vi "UHR-Fleezers Control (host) - 10.4.vi"() -> ()   [LabVIEW 2011] (continued)
            n1668 = Sign(1:w3670) -> (0:w3669:dbl)
            n1669 = Compound Arithmetic op=MULTIPLY(w3670, "MCL Step Position Ratio", "MCL/AOM Scale Tweak") -> (w3674:dbl)
            n1670 = Negate(x=w3669) -> (-x=w3666:dbl)
            n1671 = Multiply(x=w3666, y="MCL Step Increment (V_int)") -> (x*y=w3668:dbl)
            n1672 = Divide(x=w3674, y="MCL X Cal (nm/V)") -> (x/y=w3680:dbl)
            n1673 = Multiply(x=32767.0 ("y"), y=w3680) -> (x*y=w3686:dbl)
            n1674 = local read "Total Counts (ticks)"() -> (w3671:u32)
            n1675 = local read "Cycles/step (AOD)"() -> (w3682:u64)
            n1676 = local read "Scan steps (AOD)"() -> (w3683:u64)
            n1677 = Divide(x=w3686, y=10.0) -> (x/y=w3679:dbl)
            n1678 = Divide(x=w3679, y="MCL Step Increment (V_int)") -> (x/y=w3677:dbl)
            n1679 = Absolute Value(x=w3677) -> (abs(x)=w3665:dbl)
            n1680 = Compound Arithmetic op=MULTIPLY(w3683, w3682, w3671) -> (w3678:u64)
            n1681 = local write "wait to reset values"(w3693) -> ()
            n1682 = local write "MCL Scanning"(w3693) -> ()
            n1683 = Divide(x=w3678, y=w3665) -> (x/y=w3675:dbl)
            "MCL Count" <- w3675
            n1684 = xnode "Read/Write Control"("FPGA VI Reference In"=w3692, "error in"=w3691, "Scan steps (MCL)"=w3665, "Number of scans (MCL)"=w3687, "Cycles per step (MCL)"=u64 1, "Scan freq.  increment (MCL)"=w3668, "1D or 2D Scan?"=w3688, "MCL Scan Axis"=w3688, "Cont. Scan (MCL)"=w3688, "MCL count"=w3675) -> ("FPGA VI Reference Out"=w3690:T19, "error out"=w3689:errorcluster)
            n1685 = xnode "Read/Write Control"("FPGA VI Reference In"=w3690, "error in"=w3689, "AI to FIFO"=w3693, "APD to FIFO"=w3693, "Start scan"=w3693, "Start scan (MCL)"=w3693) -> ("FPGA VI Reference Out"=w3695:T19, "error out"=w3694:errorcluster)
          }
        }
        "Raster Scanning..." <- TRUE ("Scanning...")
      }
    }
    n1686 = And(x="Save scans", y=w2773) -> (x .and. y?=w2819:bool)
    n1687 = Compound Arithmetic op=OR("Start MCL Scan", "Confocal Image", "Confocal Linescan") -> (w2771:bool)
    n1688 = And(x="Save Data (MCL)", y=w2771) -> (x .and. y?=w2818:bool)
    n1689 = case "Start MCL raster scan" shown="True" w2771 {
      tunnel: w2821 -> [w3266 w3282]
      tunnel: w2820 -> [w3265 w3281]
      tunnel: [w3266 w3277] -> w2660
      tunnel: [w3265 w3276] -> w2659
      tunnel: [FALSE w3275] -> w2804
      tunnel: "Start MCL Scan" -> [_ w3270]
      tunnel: "Confocal Image" -> [_ w3269]
      tunnel: "Confocal Linescan" -> [_ _]
      frame False {
      }
      frame True {
        w3275 = TRUE
        n1690 = case shown="True" "Restart DMA? (MCL)" {
          tunnel: [w3327 w3329] -> w3280
          tunnel: [w3326 w3328] -> w3279
          tunnel: w3282 -> [w3327 w3332]
          tunnel: w3281 -> [w3326 w3331]
          frame False {
          }
          frame True {
            n1691 = call "reset FPGA DMA.vi"("error in"=w3331, "FPGA VI Reference In"=w3332) -> ("error out"=w3328:errorcluster, "FPGA VI Reference Out"=w3329:T19)
            n1692 = local write "Overflow (data lost)"(FALSE ("Overflow (data lost)")) -> ()
          }
        }
        n1693 = case shown="False" w3270 {
          selector: w3270 -> [_ w3286]
          tunnel: w3269 -> [w3285 _]
          tunnel: [w3285 w3286] -> w3268
          frame False {
            n1694 = property on="2D or 1D Scan" class="Bool (strict)"("Val(Sgnl)"=w3285) -> ()  [unwired: 2 in, 2 out]
            n1695 = property on="Confocal Image" class="Bool (strict)"("Value"=FALSE ("Start Confocal Map")) -> ()  [unwired: 2 in, 2 out]
          }
          frame True {
          }
        }
        n1696 = local write "MCL Scanning"(w3275) -> ()
        n1697 = local read "AO1"() -> (w3272:dbl)
        n1698 = local read "AO2"() -> (w3271:dbl)
        n1699 = case shown="True" "Center Scan" {
          tunnel: w3280 -> [w3293 w3325]
          tunnel: w3279 -> [w3292 w3324]
          tunnel: [w3291 w3323] -> w3277
          tunnel: [w3290 w3322] -> w3276
          tunnel: [w3288 w3309] -> w3274
          tunnel: [w3287 w3308] -> w3273
          tunnel: w3272 -> [w3288 w3314]
          tunnel: w3271 -> [w3287 w3317]
          tunnel: w3268 -> [_ _]
          frame False {
            w3289 = TRUE ("AI to FIFO")
            n1700 = xnode "Read/Write Control"("FPGA VI Reference In"=w3293, "error in"=w3292, "AI to FIFO"=w3289, "APD to FIFO"=w3289, "Start scan (MCL)"=w3289) -> ("FPGA VI Reference Out"=w3291:T19, "error out"=w3290:errorcluster)
          }
          frame True {
            w3321 = TRUE ("AI to FIFO")
            n1701 = local read "Scan steps (MCL)"() -> (w3300:u64)
            n1702 = local read "Scan lines (y)"() -> (w3296:u64)
            n1703 = local read "Fast Scan Dir"() -> (w3307:bool)
            n1704 = local read "Actual MCL Inc (V)"() -> (w3297:dbl)
            n1705 = Decrement(x=w3296) -> (x-1=w3295:u64)
            n1706 = Decrement(x=w3300) -> (x-1=w3299:u64)
            n1707 = Multiply(x=w3297, y=w3295) -> (x*y=w3294:dbl)
            n1708 = Divide(x=w3294, y=2.0) -> (x/y=w3304:dbl)
            n1709 = Multiply(x=w3297, y=w3299) -> (x*y=w3298:dbl)
            n1710 = Divide(x=w3298, y=2.0) -> (x/y=w3303:dbl)
            n1711 = Select(t=w3303, s=w3307, f=w3304) -> (s? t:f=w3302:dbl)
            n1712 = Select(t=w3304, s=w3307, f=w3303) -> (s? t:f=w3306:dbl)
            n1713 = Subtract(x=w3314, y=w3306) -> (x-y=w3305:dbl)
            n1714 = Subtract(x=w3317, y=w3302) -> (x-y=w3301:dbl)
            n1715 = local read "2D or 1D Scan"() -> (w3319:bool)
            n1716 = Not(x=w3307) -> (.not. x?=w3313:bool)
            n1717 = Not(x=w3319) -> (.not. x?=w3315:bool)
            n1718 = And(x=w3307, y=w3315) -> (x .and. y?=w3316:bool)
            n1719 = And(x=w3315, y=w3313) -> (x .and. y?=w3318:bool)
            n1720 = Select(t=w3317, s=w3318, f=w3301) -> (s? t:f=w3308:dbl)
            n1721 = Select(t=w3314, s=w3316, f=w3305) -> (s? t:f=w3309:dbl)
            n1722 = call "Volt to I16.vi"("Voltage In"=w3309) -> ("I16 Voltage Out"=w3312:i16)
            n1723 = call "Volt to I16.vi"("Voltage In"=w3308) -> ("I16 Voltage Out"=w3311:i16)
            n1724 = xnode "Read/Write Control"("FPGA VI Reference In"=w3325, "error in"=w3324, "AI to FIFO"=w3321, "APD to FIFO"=w3321, "Start scan (MCL)"=w3321, "AO1"=w3312, "AO2"=w3311) -> ("FPGA VI Reference Out"=w3323:T19, "error out"=w3322:errorcluster)
          }
        }
        "Initial Y" <- w3274
        "Initial X" <- w3273
        n1725 = local write "Tab Control 6"(T3."Imaging" ("Tab Control 6")) -> ()
        "wait to reset values" <- w3275
      }
    }
    n1726 = local read "Trap Pos Elements/DMA read"() -> (w2656:u32)
    n1727 = local read "Trap AI Elements/DMA read"() -> (w2732:u32)
    n1728 = local read "APD Elements/DMA read"() -> (w2697:u32)
    n1729 = xnode "Get APD Data"("FPGA VI Reference In"=w2660, "error in"=w2659, "Number of Elements"=w2697, "Timeout (ms)"=-1) -> ("Data"=w2696:u32[], "Elements Remaining"=→"APD FIFO Elements Remaining":u32)  [unwired: 2 out]
    n1730 = xnode "Invoke Method"("FPGA VI Reference In"=w2660, "error in"=w2659, "Number of Elements"=w2656, "Timeout (ms)"=-1) -> ("Data"=w2619:u16[], "Elements Remaining"=→"Trap Pos FIFO El Remaining":u32)  [unwired: 2 out]
    n1731 = xnode "Get Trap Data"("FPGA VI Reference In"=w2660, "error in"=w2659, "Number of Elements"=w2732, "Timeout (ms)"=-1 ("Timeout")) -> ("FPGA VI Reference Out"=w2553:T19, "error out"=w2552:errorcluster, "Data"=w2620:i16[], "Elements Remaining"=w2865:u32)
    "FIFO El. Rem." <- w2865
    n1732 = local read "Trap AI FIFO Depth"() -> (w2867:u32)
    n1733 = Subtract(x=w2867, y=w2732) -> (x-y=w2866:u32)
    n1734 = Decimate 1D Array(w2619) -> (w2616:u16[], w2618:u16[], w2617:u16[])
    n1735 = Divide(x=w2865, y=w2866) -> (x/y=w2864:dbl)
    "Buffer Status" <- w2864
    n1736 = To Unsigned Long Integer(number=w2616) -> (unsigned 32bit integer=w2615:u32[])
    n1737 = Join Numbers(hi=w2618, lo=w2617) -> ((hi.lo)=w2614:u32[])
    n1738 = Equal?(x=w2864, y=1.0) -> (x = y?=w2862:bool)
    n1739 = Join Numbers(hi=w2615, lo=w2614) -> ((hi.lo)=w2608:u64[])
    n1740 = call "IR AOM word to freq - vec.vi"("Frequency Word In (double vec)"=w2608) -> ("Frequency Out"=w2655:dbl[])
    n1741 = case "Alert buffer overflow" shown="True" w2862 {
      frame False {
      }
      frame True {
        n1742 = call <vilib>:"Beep.vi"() -> ()  [unwired: 3 in, 9 out]
        "Overflow (data lost)" <- TRUE ("Overflow (data lost)")
      }
    }
    n1743 = Decimate 1D Array(w2655) -> (w2654:dbl[], w2653:dbl[])
    n1744 = Build Array(w2654, w2653) -> (w2652:dbl[][])
    n1745 = local read "Trap Sets"() -> (w2731:u32)
    n1746 = case "Deinterlace trap data, average down PSD" shown="2" w2731 {
      tunnel: w2620 -> [w3362 w3427]
      tunnel: [w3359 w3424] -> w2724
      tunnel: [w3362 w3426] -> w2611
      tunnel: "Detector Type" -> [w3361 w3422]
      tunnel: [w3360 w3425] -> w2723
      tunnel: [w3358 w3423] -> w2839
      frame 1, Default {
        n1747 = Divide(x=w3362, y=3276.7) -> (x/y=w3363:dbl[])
        n1748 = Decimate 1D Array(w3363) -> (w3372:dbl[], w3371:dbl[], w3370:dbl[], w3369:dbl[], w3368:dbl[], w3367:dbl[], w3366:dbl[], w3365:dbl[])
        n1749 = case shown="\"IR-QPD + PSD + FB-QPD position\"" w3361 {
          tunnel: w3372 -> [w3396 w3421]
          tunnel: w3371 -> [w3395 w3420]
          tunnel: w3370 -> [w3380 w3398]
          tunnel: w3369 -> [w3381 w3408]
          tunnel: w3368 -> [w3394 w3419]
          tunnel: w3367 -> [w3393 w3418]
          tunnel: w3366 -> [w3377 w3399]
          tunnel: w3365 -> [w3376 w3397]
          tunnel: [w3375 w3405] -> w3360
          tunnel: [w3374 w3404] -> w3359
          tunnel: [w3373 w3403] -> w3358
          frame "IR-QPD + PSD + FB-QPD", Default {
            w3373 = 0  # Channel pattern
            n1750 = Divide(x=w3396, y=w3381) -> (x/y=w3383:dbl[])
            n1751 = Divide(x=w3395, y=w3381) -> (x/y=w3382:dbl[])
            n1752 = Divide(x=w3394, y=w3377) -> (x/y=w3379:dbl[])
            n1753 = Divide(x=w3393, y=w3376) -> (x/y=w3378:dbl[])
            n1754 = Build Array(w3383, w3382, w3381, w3380, w3379, w3378, w3377, w3376) -> (w3374:dbl[][])
            n1755 = Bundle("T1 Y", "T1 X", "T1 Sum", "FB Sum", "PSD Y", "PSD X", "PSD Y Sum", "PSD X Sum") -> (w3392:T40)  [unwired: 1 out]
            n1756 = Cluster To Array(cluster=w3392) -> (array=w3375:string[])
          }
          frame "IR-QPD + PSD + FB-QPD position" {
            w3403 = 3  # Channel pattern
            n1757 = Negate(x=w3399) -> (-x=w3400:dbl[])
            n1758 = Divide(x=w3421, y=w3408) -> (x/y=w3410:dbl[])
            n1759 = Divide(x=w3420, y=w3408) -> (x/y=w3409:dbl[])
            n1760 = Divide(x=w3419, y=w3399) -> (x/y=w3407:dbl[])
            n1761 = Divide(x=w3418, y=w3400) -> (x/y=w3406:dbl[])
            n1762 = Build Array(w3410, w3409, w3408, w3397, w3398, w3407, w3406, w3399) -> (w3404:dbl[][])
            n1763 = Bundle("T1 Y", "T1 X", "T1 Sum", "FB X", "FB Sum", "PSD Y", "PSD X", "PSD Y Sum") -> (w3417:T40)  [unwired: 1 out]
            n1764 = Cluster To Array(cluster=w3417) -> (array=w3405:string[])
          }
        }
      }
      frame 2 {
        n1765 = case shown="\"IR-QPD + PSD + FB-QPD X position\"" w3422 {
          tunnel: w3427 -> [w3489 w3556 w3627]
          tunnel: [w3428 w3547 w3558] -> w3426
          tunnel: [w3455 w3538 w3605] -> w3425
          tunnel: [w3454 w3501 w3572] -> w3424
          tunnel: [w3448 w3536 w3603] -> w3423
          frame "IR-QPD + PSD + FB-QPD", Default {
            w3448 = 1  # Channel pattern
            # "time average x2 the 4th signal and the 4 psd signals (detection laser)"
            # "deinterlace 3 signals from qpd"
            n1766 = Decimate 1D Array(w3489) -> (w3488:i16[], w3487:i16[], w3453:i16[], w3486:i16[], w3476:i16[], w3474:i16[], w3473:i16[], w3471:i16[])
            n1767 = Decimate 1D Array(w3453) -> (w3452:i16[], w3451:i16[])
            n1768 = Decimate 1D Array(w3488) -> (w3485:i16[], w3457:i16[])
            n1769 = Decimate 1D Array(w3487) -> (w3484:i16[], w3482:i16[])
            n1770 = Decimate 1D Array(w3486) -> (w3483:i16[], w3481:i16[])
            n1771 = call "downsample 1D array - double.vi"("Ave N"=2.0, "Array In"=w3476) -> ("Array Out"=w3475:dbl[])  [unwired: 1 out]
            n1772 = call "downsample 1D array - double.vi"("Ave N"=2.0, "Array In"=w3474) -> ("Array Out"=w3456:dbl[])  [unwired: 1 out]
            n1773 = call "downsample 1D array - double.vi"("Ave N"=2.0, "Array In"=w3473) -> ("Array Out"=w3472:dbl[])  [unwired: 1 out]
            n1774 = call "downsample 1D array - double.vi"("Ave N"=2.0, "Array In"=w3471) -> ("Array Out"=w3470:dbl[])  [unwired: 1 out]
            n1775 = Interleave 1D Arrays(w3485, w3484, w3483, w3457, w3482, w3481, w3452, w3451, w3475, w3456, w3472, w3470) -> (w3469:dbl[])
            n1776 = Divide(x=w3469, y=3276.7) -> (x/y=w3468:dbl[])
            n1777 = Decimate 1D Array(w3468) -> (w3467:dbl[], w3466:dbl[], w3465:dbl[], w3464:dbl[], w3463:dbl[], w3462:dbl[], w3450:dbl[], w3449:dbl[], w3461:dbl[], w3460:dbl[], w3459:dbl[], w3458:dbl[])
            n1778 = Divide(x=w3467, y=w3465) -> (x/y=w3435:dbl[])
            n1779 = Divide(x=w3466, y=w3465) -> (x/y=w3434:dbl[])
            n1780 = Divide(x=w3464, y=w3462) -> (x/y=w3433:dbl[])
            n1781 = Divide(x=w3463, y=w3462) -> (x/y=w3432:dbl[])
            n1782 = Divide(x=w3461, y=w3459) -> (x/y=w3431:dbl[])
            n1783 = Divide(x=w3460, y=w3458) -> (x/y=w3430:dbl[])
            n1784 = Build Array(w3435, w3434, w3465, w3433, w3432, w3462, w3450, w3449, w3431, w3430, w3459, w3458) -> (w3454:dbl[][])
            n1785 = Bundle("T1 Y", "T1 X", "T1 Sum", "T2 Y", "T2 X", "T2 Sum", "T1 FB Sum", "T2 FB Sum", "PSD Y", "PSD X", "PSD Y Sum", "PSD X Sum") -> (w3436:T41)  [unwired: 1 out]
            n1786 = To Word Integer(number=w3469) -> (16bit integer=w3428:i16[])
            n1787 = Cluster To Array(cluster=w3436) -> (array=w3455:string[])
          }
          frame "IR-QPD + PSD + FB-QPD X position" {
            w3536 = 2  # Channel pattern
            # "time average x2 the 3 psd signals (detection laser)"
            # "deinterlace 3 signals from qpds"
            n1788 = Decimate 1D Array(w3556) -> (w3555:i16[], w3554:i16[], w3537:i16[], w3553:i16[], w3499:i16[], w3496:i16[], w3493:i16[], w3524:i16[])
            n1789 = Decimate 1D Array(w3537) -> (w3522:i16[], w3520:i16[])
            n1790 = Decimate 1D Array(w3555) -> (w3552:i16[], w3539:i16[])
            n1791 = Decimate 1D Array(w3554) -> (w3551:i16[], w3549:i16[])
            n1792 = Decimate 1D Array(w3553) -> (w3550:i16[], w3548:i16[])
            n1793 = Decimate 1D Array(w3524) -> (w3523:i16[], w3521:i16[])
            n1794 = call "downsample 1D array - I16.vi"("Ave N"=2.0, "Array In"=w3499) -> ("Array Out"=w3497:i16[])  [unwired: 1 in]
            n1795 = call "downsample 1D array - I16.vi"("Ave N"=2.0, "Array In"=w3493) -> ("Array Out"=w3491:i16[])  [unwired: 1 in]
            n1796 = call "downsample 1D array - I16.vi"("Ave N"=2.0, "Array In"=w3496) -> ("Array Out"=w3494:i16[])  [unwired: 1 in]
            n1797 = Interleave 1D Arrays(w3552, w3551, w3550, w3539, w3549, w3548, w3523, w3522, w3521, w3520, w3497, w3494, w3491) -> (w3547:i16[])
            n1798 = Divide(x=w3547, y=3276.7) -> (x/y=w3546:dbl[])
            n1799 = Decimate 1D Array(w3546) -> (w3545:dbl[], w3544:dbl[], w3543:dbl[], w3542:dbl[], w3541:dbl[], w3540:dbl[], w3512:dbl[], w3510:dbl[], w3509:dbl[], w3507:dbl[], w3506:dbl[], w3505:dbl[], w3502:dbl[])
            n1800 = Negate(x=w3502) -> (-x=w3500:dbl[])
            n1801 = Divide(x=w3506, y=w3502) -> (x/y=w3504:dbl[])
            n1802 = Divide(x=w3505, y=w3500) -> (x/y=w3503:dbl[])
            n1803 = Divide(x=w3545, y=w3543) -> (x/y=w3528:dbl[])
            n1804 = Divide(x=w3544, y=w3543) -> (x/y=w3527:dbl[])
            n1805 = Divide(x=w3542, y=w3540) -> (x/y=w3526:dbl[])
            n1806 = Divide(x=w3541, y=w3540) -> (x/y=w3525:dbl[])
            n1807 = Divide(x=w3512, y=w3510) -> (x/y=w3511:dbl[])
            n1808 = Divide(x=w3509, y=w3507) -> (x/y=w3508:dbl[])
            n1809 = Build Array(w3528, w3527, w3543, w3526, w3525, w3540, w3511, w3510, w3508, w3507, w3504, w3503, w3502) -> (w3501:dbl[][])
            n1810 = Bundle("T1 Y", "T1 X", "T1 Sum", "T2 Y", "T2 X", "T2 Sum", "T1 FB X", "T1 FB Sum", "T2 FB X", "T2 FB Sum", "PSD Y", "PSD X", "PSD Y Sum") -> (w3529:T42)  [unwired: 1 out]
            n1811 = Cluster To Array(cluster=w3529) -> (array=w3538:string[])
          }
          frame "IR-QPD + PSD + FB-QPD XY positions" {
            w3603 = 4  # Channel pattern
            # "time average x2 the 3 psd signals (detection laser)"
            # "deinterlace 3 signals from qpds"
            n1812 = Decimate 1D Array(w3627) -> (w3626:i16[], w3625:i16[], w3604:i16[], w3624:i16[], w3570:i16[], w3616:i16[], w3615:i16[], w3592:i16[])
            n1813 = Decimate 1D Array "Feedback Sum"(w3604) -> (w3588:i16[], w3586:i16[])
            n1814 = Decimate 1D Array "QPD Y"(w3626) -> (w3623:i16[], w3606:i16[])
            n1815 = Decimate 1D Array "QPD X"(w3625) -> (w3622:i16[], w3620:i16[])
            n1816 = Decimate 1D Array "Feedback Y"(w3570) -> (w3569:i16[], w3568:i16[])
            n1817 = Decimate 1D Array "QPD Sum"(w3624) -> (w3621:i16[], w3619:i16[])
            n1818 = Decimate 1D Array "Feedback X"(w3592) -> (w3589:i16[], w3587:i16[])
            n1819 = call "downsample 1D array - double.vi"("Ave N"=2.0, "Array In"=w3616) -> ("Array Out"=w3591:dbl[])  [unwired: 1 out]
            n1820 = call "downsample 1D array - double.vi"("Ave N"=2.0, "Array In"=w3615) -> ("Array Out"=w3590:dbl[])  [unwired: 1 out]
            n1821 = Interleave 1D Arrays(w3623, w3622, w3621, w3606, w3620, w3619, w3569, w3589, w3588, w3568, w3587, w3586, w3591, w3590) -> (w3614:dbl[])
            n1822 = Divide(x=w3614, y=3276.7) -> (x/y=w3613:dbl[])
            n1823 = Decimate 1D Array(w3613) -> (w3612:dbl[], w3611:dbl[], w3610:dbl[], w3609:dbl[], w3608:dbl[], w3607:dbl[], w3565:dbl[], w3579:dbl[], w3563:dbl[], w3564:dbl[], w3577:dbl[], w3561:dbl[], w3575:dbl[], w3573:dbl[])
            n1824 = Negate(x=w3573) -> (-x=w3571:dbl[])
            n1825 = Divide(x=w3575, y=w3571) -> (x/y=w3574:dbl[])
            n1826 = Divide(x=w3564, y=w3561) -> (x/y=w3560:dbl[])
            n1827 = Divide(x=w3565, y=w3563) -> (x/y=w3562:dbl[])
            n1828 = Divide(x=w3612, y=w3610) -> (x/y=w3596:dbl[])
            n1829 = Divide(x=w3611, y=w3610) -> (x/y=w3595:dbl[])
            n1830 = Divide(x=w3609, y=w3607) -> (x/y=w3594:dbl[])
            n1831 = Divide(x=w3608, y=w3607) -> (x/y=w3593:dbl[])
            n1832 = Divide(x=w3579, y=w3563) -> (x/y=w3578:dbl[])
            n1833 = Divide(x=w3577, y=w3561) -> (x/y=w3576:dbl[])
            n1834 = Build Array(w3596, w3595, w3610, w3594, w3593, w3607, w3562, w3578, w3563, w3560, w3576, w3561, w3574, w3573) -> (w3572:dbl[][])
            n1835 = Bundle("T1 Y", "T1 X", "T1 Sum", "T2 Y", "T2 X", "T2 Sum", "T1 FB Y", "T1 FB X", "T1 FB Sum", "T2 FB Y", "T2 FB X", "T2 FB Sum", "PSD X", "PSD Y Sum") -> (w3559:T43)  [unwired: 1 out]
            n1836 = To Word Integer(number=w3614) -> (16bit integer=w3558:i16[])
            n1837 = Cluster To Array(cluster=w3559) -> (array=w3605:string[])
          }
        }
      }
    }
    "AI labels" <- w2723
    n1838 = Decimate 1D Array(w2696) -> (w2721:u32[], w2664:u32[])
    n1839 = local read "DMA Update Period (s)"() -> (w2733:dbl)
    n1840 = Build Array(w2721, w2664) -> (w2801:u32[][])
    n1841 = local read "Data Period (s)"() -> (w2570:dbl)
    n1842 = local read "BD 1 Frequency 2 (MHz)"() -> (w2603:dbl)
    n1843 = local read "BD 1 Frequency 1 (MHz)"() -> (w2604:dbl)
    n1844 = Decimate 1D Array(w2611) -> (w2635:i16[], w2634:i16[], w2632:i16[], w2631:i16[])  [unwired: 9 out]
    n1845 = To Double Precision Float(number=w2801) -> (double precision float=w2802:dbl[][])
    n1846 = local read "APD Integration Time (s)"() -> (w2677:dbl)
    n1847 = Multiply(x=w2570, y="Trap Pos. Disp. Downsample") -> (x*y=w2568:dbl)
    n1848 = Divide(x=w2635, y=w2634) -> (x/y=w2636:dbl[])
    n1849 = Divide(x=w2632, y=w2631) -> (x/y=w2633:dbl[])
    n1850 = feedback #4(0.0) -> (w2649:dbl)
    n1851 = Add(x=w2733, y=w2649) -> (x+y=w2841:dbl)
    n1852 = feedback-in #4(w2841) -> ()
    n1853 = local read "AOM X Cal (nm/MHz)"() -> (w2601:dbl)
    n1854 = To Time Stamp(1:w2649) -> (0:w2648:timestamp)
    n1855 = Split 1D Array(array=w2636, index="N El. to Ave.") -> (second subarray=w2639:dbl[])  [unwired: 1 out]
    n1856 = Split 1D Array(array=w2633, index="N El. to Ave.") -> (second subarray=w2638:dbl[])  [unwired: 1 out]
    n1857 = Multiply(x=w2570, y="Trap Disp. Downsample") -> (x*y=w2650:dbl)
    "Display Period (s)" <- w2650
    n1858 = for "Trap AI" {
      tunnel: [w3357] -> w2835 mode=indexing
      tunnel: w2648 -> [w3347]
      tunnel: "Trap Disp. Downsample" -> [w3355]
      tunnel: w2724 -> [w3353] mode=indexing
      tunnel: w2570 -> [w3352]
      tunnel: w2723 -> [w3351] mode=indexing
      tunnel: w2647 -> [w3350]
      tunnel: [w3349] -> w2688 mode=indexing
      tunnel: w2650 -> [w3348]
      workers-P: _ -> [_]
      n1859 = Bundle By Name("Y"=w3353, "dt"=w3352) -> (w3354:waveform(dbl))  [unwired: 1 out]
      n1860 = Set Waveform Attribute(5:w3351, 6:w3350, 7:w3354) -> (3:w3349:waveform(dbl))  [unwired: 1 in, 2 out]
      n1861 = call "downsample 1D array - double.vi"("Ave N"=w3355, "Array In"=w3353) -> ("Array Out"=w3356:dbl[])  [unwired: 1 out]
      n1862 = Bundle By Name(cluster=w3349, "t0"=w3347, "Y"=w3356, "dt"=w3348) -> (w3357:waveform(dbl))
    }
    n1863 = Bundle("BD 1 Frequency 1 (MHz)"=w2604, "BD 1 Frequency 2 (MHz)"=w2603) -> (w2605:T44)  [unwired: 1 out]
    n1864 = call <vilib>:"Mean.vi"("X"=w2638) -> ("mean"=w2626:dbl)  [unwired: 1 out]
    n1865 = call <vilib>:"Mean.vi"("X"=w2639) -> ("mean"=w2627:dbl)  [unwired: 1 out]
    n1866 = Reciprocal(x=w2650) -> (1/x=→"Trap Disp. Freq. (Hz)":dbl)
    n1867 = Cluster To Array(cluster=w2605) -> (array=w2602:dbl[])
    n1868 = local read "Trap X AI1 (DMA)"() -> (w2637:T13)
    n1869 = local read "Data points/scans (MCL)"() -> (w2813:dbl)
    n1870 = To Fixed-Point(number=w2626) -> (fixed-point=w2624:fxp<+/-,16,1>)  [unwired: 1 in]
    n1871 = To Fixed-Point(number=w2627) -> (fixed-point=w2625:fxp<+/-,16,1>)  [unwired: 1 in]
    n1872 = Bundle("Trap 1 Pos.", "Trap 2 Pos.") -> (w2646:cluster{string, string})  [unwired: 1 out]
    n1873 = Bundle By Name(cluster=w2637, "Set 1"=w2625, "Set 2"=w2624) -> (→"Trap X AI1 (DMA)":T13)
    n1874 = Cluster To Array(cluster=w2646) -> (array=w2643:string[])
    n1875 = Bundle("APD 1", "APD 2") -> (w2834:cluster{string, string})  [unwired: 1 out]
    n1876 = Select(t=-1.0, s="Negate Y Axis", f=1.0) -> (s? t:f=w2587:dbl)
    n1877 = for "Trap Position" {
      tunnel: w2652 -> [w2996] mode=indexing
      tunnel: "Trap Pos. Disp. Downsample" -> [w2995]
      tunnel: w2568 -> [w2993]
      tunnel: w2648 -> [w2992]
      tunnel: w2647 -> [w2990]
      tunnel: w2643 -> [w2989] mode=indexing
      tunnel: [w2988] -> w2557 mode=indexing
      tunnel: w2602 -> [w2986] mode=indexing
      tunnel: w2601 -> [w2984]
      tunnel: w2587 -> [w2983]
      n1878 = call "downsample 1D array - double.vi"("Ave N"=w2995, "Array In"=w2996) -> ("Array Out"=w2994:dbl[])  [unwired: 1 out]
      n1879 = Subtract(x=w2994, y=w2986) -> (x-y=w2987:dbl[])
      n1880 = Multiply(x=w2984, y=w2987) -> (x*y=w2985:dbl[])
      n1881 = Multiply(x=w2983, y=w2985) -> (x*y=w2982:dbl[])
      n1882 = Bundle By Name("Y"=w2982, "dt"=w2993, "t0"=w2992) -> (w2991:waveform(dbl))  [unwired: 1 out]
      n1883 = Set Waveform Attribute(5:w2989, 6:w2990, 7:w2991) -> (3:w2988:waveform(dbl))  [unwired: 1 in, 2 out]
    }
    n1884 = Cluster To Array(cluster=w2834) -> (array=w2831:string[])
    n1885 = for "APD" {
      tunnel: w2802 -> [w3336] mode=indexing
      tunnel: w2677 -> [w3344]
      tunnel: [w3340] -> w2684 mode=indexing
      tunnel: "APD Disp. Scale" -> [w3341]
      tunnel: w2647 -> [w3339]
      tunnel: w2831 -> [w3338] mode=indexing
      tunnel: "APD Disp. Downsample" -> [w3334]
      tunnel: [w3337] -> w2830
      workers-P: _ -> [_]
      tunnel: w2648 -> [w3333]
      n1886 = call "integrate 1D array interval - double.vi"("Ave N"=w3334, "Array In"=w3336) -> ("Array Out"=w3335:dbl[])  [unwired: 1 out]
      n1887 = Multiply(x=w3344, y=w3334) -> (x*y=w3337:dbl)
      n1888 = Divide(x=w3335, y=w3341) -> (x/y=w3342:dbl[])
      n1889 = Bundle By Name("t0"=w3333, "Y"=w3342, "dt"=w3337) -> (w3343:waveform(dbl))  [unwired: 1 out]
      n1890 = Set Waveform Attribute(5:w3338, 6:w3339, 7:w3343) -> (3:w3340:waveform(dbl))  [unwired: 1 in, 2 out]
    }
    "APD Display Period (s)" <- w2830
    n1891 = Reciprocal(x=w2830) -> (1/x=→"APD Display Freq. (Hz)":dbl)
    n1892 = local read "Display Period (s)"() -> (w2708:dbl)
    n1893 = Increment(x=w2813) -> (x+1=w2814:dbl)
    n1894 = To Double Precision Float(number=w2721) -> (double precision float=w2720:dbl[])
    n1895 = Index Array(array=w2557, index=0) -> (element=w2561:waveform(dbl))
    n1896 = Index Array(array=w2557, index=1) -> (element=w2556:waveform(dbl))
    n1897 = feedback #5(w2814) -> (w2817:dbl)
    n1898 = Select(t=0, s=w2804, f=w2817) -> (s? t:f=w2810:dbl)
    n1899 = Array Size(array=w2720) -> (size(s)=w2816:i32)
    n1900 = Add(x=w2816, y=w2810) -> (x+y=w2811:dbl)
    n1901 = Unbundle By Name(w2561) -> ("Y"=w2562:dbl[])
    n1902 = feedback #6(w2721) -> (w2800:u32[])
    n1903 = Build Array (concatenate)(w2800, w2721) -> (w2797:u32[])
    n1904 = feedback #7(w2664) -> (w2683:u32[])
    n1905 = Divide(x="Bead Sep. Int. Time (s)", y=w2708) -> (x/y=w2597:dbl)
    n1906 = Build Array (concatenate)(w2683, w2664) -> (w2682:u32[])
    n1907 = Add(x=w2562, y="FB Trap Pos Offset") -> (x+y=w2560:dbl[])
    "T1 x pos data" <- w2560
    n1908 = Greater?(x=w2811, y=w2813) -> (0:w2812:bool)
    n1909 = feedback #8(w2560) -> (w2599:dbl[])
    n1910 = Build Array (concatenate)(w2560, w2599) -> (w2598:dbl[])
    n1911 = Bundle By Name(cluster=w2561, "Y"=w2560) -> (w2559:waveform(dbl))
    n1912 = Select(t=w2810, s=w2812, f=w2811) -> (s? t:f=w2809:dbl)
    n1913 = feedback-in #5(w2809) -> ()
    n1914 = Array Size(array=w2797) -> (size(s)=w2794:i32)
    n1915 = Array Size(array=w2721) -> (size(s)=w2796:i32)
    n1916 = local read "MCL Scanning"() -> (w2807:bool)
    n1917 = local read "APD Integration Time (s)"() -> (w2691:dbl)
    n1918 = Bundle(w2559, w2556) -> (w2555:cluster{waveform(dbl), waveform(dbl)})  [unwired: 1 out]
    n1919 = Build Array (concatenate)(w2684, w2835) -> (w2686:waveform(dbl)[])
    "All Signals" <- w2686
    n1920 = Split 1D Array(array=w2598, index=w2597) -> (first subarray=w2591:dbl[])  [unwired: 1 out]
    n1921 = feedback-in #8(w2591) -> ()
    n1922 = Multiply(x=w2796, y="APD Ave N") -> (x*y=w2795:dbl)
    n1923 = Greater?(x=w2794, y=w2795) -> (0:w2798:bool)
    n1924 = Not(x=w2812) -> (.not. x?=w2806:bool)
    n1925 = Cluster To Array(cluster=w2555) -> (array=→"Trap Positions":waveform(dbl)[])
    n1926 = To Double Precision Float(number=w2664) -> (double precision float=w2663:dbl[])
    n1927 = call <vilib>:"Mean.vi"("X"=w2591) -> ("mean"=w2590:dbl)  [unwired: 1 out]
    "Mean T1 Position (nm)" <- w2590
    n1928 = Subtract(x=w2591, y=w2590) -> (x-y=w2596:dbl[])
    n1929 = Square(x=w2596) -> (x^2=w2595:dbl[])
    n1930 = And(x=w2806, y=w2807) -> (x .and. y?=w2808:bool)
    n1931 = call <vilib>:"Mean.vi"("X"=w2595) -> ("mean"=w2594:dbl)  [unwired: 1 out]
    n1932 = case shown="True" w2798 {
      tunnel: w2797 -> [w3116 w3123]
      tunnel: [w3116 w3121] -> w2738
      tunnel: w2795 -> [_ w3118]
      tunnel: w2794 -> [_ w3122]
      tunnel: w2682 -> [w3115 w3120]
      tunnel: [w3115 w3117] -> w2679
      frame False {
      }
      frame True {
        n1933 = Subtract(x=w3122, y=w3118) -> (x-y=w3119:dbl)
        n1934 = Array Subset(array=w3123, index=w3119, length=w3118) -> (w3121:u32[])
        n1935 = Array Subset(array=w3120, index=w3119, length=w3118) -> (w3117:u32[])
      }
    }
    n1936 = feedback-in #6(w2738) -> ()
    n1937 = feedback-in #7(w2679) -> ()
    n1938 = Square Root(x=w2594) -> (sqrt(x)=w2593:dbl)
    n1939 = Or(x=w2808, y=w2804) -> (x .or. y?=w2805:bool)
    n1940 = Equal?(x="Tab Control 6", y=T34."High Res Display") -> (x = y?=w2727:bool)
    n1941 = Multiply(x="APD Disp. Scale", y=w2684) -> (x*y=w2693:waveform(dbl)[])
    n1942 = Multiply(x=10.0, y=w2593) -> (x*y=→"Trap 1 Position RMS (A)":dbl)
    n1943 = Multiply(x="APD Disp. Downsample", y=w2691) -> (x*y=w2689:dbl)
    n1944 = Divide(x=w2693, y=w2689) -> (x/y=w2661:waveform(dbl)[])
    n1945 = case "For displaying the high resolution display (no downsampling)" shown="True" w2727 {
      tunnel: w2688 -> [_ w3016]
      frame False {
      }
      frame True {
        n1946 = Index Array(array=w3016, index="High Res. Display") -> (element=w3017:waveform(dbl))
        n1947 = call <vilib>:"Std Deviation and Variance.vi"("X"=w3017) -> ("mean"=w3024:dbl, "standard deviation"=w3029:dbl)  [unwired: 1 in, 1 out]
        "Mean Intensity" <- w3024
        "Sigma" <- w3029
        n1948 = Subtract(x=w3017, y=w3024) -> (x-y=w3023:waveform(dbl))
        n1949 = Select(t=w3023, s="Subtract mean", f=w3017) -> (s? t:f=→"1 Channel":waveform(dbl))
        n1950 = Divide(x=w3029, y=w3024) -> (x/y=→"Sigma/Mean":dbl)
        n1951 = feedback #9(1) -> (w3018:i32)
        n1952 = Greater Or Equal?(x=w3018, y="Slow mean N ave.") -> (x >= y?=w3031:bool)
        n1953 = Increment(x=w3018) -> (x+1=w3033:i32)
        n1954 = Select(t=1, s=w3031, f=w3033) -> (s? t:f=w3020:i32)
        n1955 = feedback-in #9(w3020) -> ()
        n1956 = feedback #10() -> (w3021:waveform(dbl))  [unwired: 1 out]
        n1957 = case shown="Default" w3018 {
          tunnel: [w3036 w3039] -> w3022
          tunnel: w3021 -> [w3038 _]
          tunnel: w3017 -> [w3037 w3039]
          frame Default {
            n1958 = call-poly <vilib>:"Append Waveforms.vi"("waveform B"=w3037, "waveform A"=w3038) -> ("waveform out"=w3036:waveform(dbl))  [unwired: 1 in, 8 out]
          }
          frame 1 {
          }
        }
        n1959 = feedback-in #10(w3022) -> ()
        n1960 = case shown="True" w3031 {
          tunnel: w3022 -> [_ w3035]
          frame False {
          }
          frame True {
            n1961 = call <vilib>:"Mean.vi"("X"=w3035) -> ("mean"=→"Slow mean":dbl)  [unwired: 1 out]
          }
        }
      }
    }
    n1962 = Index Array(array=w2661, index=0) -> (element=w2671:waveform(dbl))
    n1963 = Index Array(array=w2661, index=1) -> (element=w2669:waveform(dbl))
    n1964 = case "For computing FFTs for display" shown="True" "Compute FFT" {
      tunnel: w2688 -> [_ w3730]
      frame False {
      }
      frame True {
        n1965 = Build Array("FFT 1 Choice 1", "FFT 1 Choice 2", "FFT 2 Choice 1", "FFT 2 Choice 2") -> (w3723:u16[])
        n1966 = Array Size(array=w3730) -> (size(s)=w3729:i32)
        n1967 = feedback-in #11(w3723) -> ()
        n1968 = feedback #11(u16[] [100, 100, 100, 100]) -> (w3724:u16[])
        n1969 = feedback-in #12("# Spectra to Ave.") -> ()
        n1970 = feedback #12("# Spectra to Ave.") -> (w3721:dbl)
        n1971 = Not Equal?(x="# Spectra to Ave.", y=w3721) -> (x != y?=w3720:bool)
        n1972 = Not Equal?(x=w3723, y=w3724) -> (x != y?=w3722:bool)
        n1973 = feedback #13(1.0) -> (w3707:dbl)
        n1974 = Compound Arithmetic op=OR("Reset FFT", w3722, w3720) -> (w3705:bool)
        n1975 = Select(t=1.0, s=w3705, f=w3707) -> (s? t:f=w3709:dbl)
        n1976 = Greater?(x=w3709, y="# Spectra to Ave.") -> (0:w3728:bool)
        n1977 = Increment(x=w3709) -> (x+1=w3708:dbl)
        n1978 = feedback-in #13(w3708) -> ()
        n1979 = local read "DMA Update Period (s)"() -> (w3703:dbl)
        n1980 = Multiply(x="# Spectra to Ave.", y=w3703) -> (x*y=→"Ave. Time (s)":dbl)
        n1981 = Build Array(cluster{"f0":dbl, "df":dbl, "magnitude":dbl[]} {"f0"=0.0, "df"=0.0, "magnitude"=[]} ("PSD")) -> (w3712:cluster{"f0":dbl, "df":dbl, "magnitude":dbl[]}[])
        n1982 = Build Array(w3712, w3712, w3712, w3712) -> (w3714:T45)
        n1983 = feedback #14(w3714) -> (w3719:T45)
        n1984 = for {
          N: 4 -> [_]
          tunnel: w3723 -> [w3752] mode=indexing
          tunnel: w3730 -> [w3753]
          tunnel: w3729 -> [w3755]
          tunnel: w3705 -> [w3748]
          tunnel: w3728 -> [w3747]
          tunnel: "# Spectra to Ave." -> [w3746]
          tunnel: [w3745] -> w3718 mode=indexing
          tunnel: w3719 -> [w3750] mode=indexing
          tunnel: [w3749] -> w3706 mode=indexing
          tunnel: w3709 -> [w3744]
          n1985 = Less?(x=w3752, y=w3755) -> (x < y?=w3754:bool)
          n1986 = Index Array(array=w3753, index=w3752) -> (element=w3751:waveform(dbl))
          n1987 = case shown="True" w3754 {
            tunnel: w3751 -> [_ w3772]
            tunnel: w3750 -> [w3757 w3770]
            tunnel: [w3757 w3758] -> w3749
            tunnel: w3748 -> [_ w3769]
            tunnel: w3747 -> [_ w3762]
            tunnel: w3746 -> [_ w3761]
            tunnel: [cluster{"f0":dbl, "df":dbl, "magnitude":dbl[]} {"f0"=0.0, "df"=0.0, "magnitude"=[]} ("PSD") w3763] -> w3745
            tunnel: w3744 -> [_ w3760]
            frame False {
            }
            frame True {
              n1988 = call <vilib>:"Std Deviation and Variance.vi"("X"=w3772) -> ("mean"=w3773:dbl)  [unwired: 1 in, 2 out]
              n1989 = Subtract(x=w3772, y=w3773) -> (x-y=w3771:waveform(dbl))
              n1990 = xnode "Spectral Measurements"("Signals"=w3771) -> ("PSD"=w3765:cluster{"f0":dbl, "df":dbl, "magnitude":dbl[]})  [unwired: 1 in, 1 out]
              n1991 = case shown="False" w3769 {
                tunnel: w3770 -> [w3782 _]
                tunnel: [w3778 w3787] -> w3758
                tunnel: w3765 -> [w3781 w3788]
                tunnel: w3762 -> [w3780 _]
                frame False {
                  n1992 = Build Array (concatenate)(w3782, w3781) -> (w3779:cluster{"f0":dbl, "df":dbl, "magnitude":dbl[]}[])
                  n1993 = case shown="True" w3780 {
                    tunnel: w3779 -> [w3783 w3786]
                    tunnel: [w3783 w3784] -> w3778
                    frame False {
                    }
                    frame True {
                      n1994 = Delete From Array(array=w3786, index=0) -> (array with subset deleted=w3784:cluster{"f0":dbl, "df":dbl, "magnitude":dbl[]}[])  [unwired: 1 in, 1 out]
                    }
                  }
                }
                frame True {
                  n1995 = Build Array(w3788) -> (w3787:cluster{"f0":dbl, "df":dbl, "magnitude":dbl[]}[])
                }
              }
              n1996 = for {
                tunnel: w3758 -> [w3777] mode=indexing
                tunnel: [w3776] -> w3768 mode=indexing
                workers-P: _ -> [_]
                n1997 = Unbundle By Name(w3777) -> ("magnitude"=w3776:dbl[])
              }
              n1998 = Transpose 2D Array(2D array=w3768) -> (transposed array=w3767:dbl[][])
              n1999 = for {
                tunnel: w3767 -> [w3775] mode=indexing
                tunnel: [w3774] -> w3766 mode=indexing
                workers-P: _ -> [_]
                n2000 = Add Array Elements(numeric array=w3775) -> (sum=w3774:dbl)
              }
              n2001 = Select(t=w3761, s=w3762, f=w3760) -> (s? t:f=w3759:dbl)
              n2002 = Divide(x=w3766, y=w3759) -> (x/y=w3764:dbl[])
              n2003 = Bundle By Name(cluster=w3765, "magnitude"=w3764) -> (w3763:cluster{"f0":dbl, "df":dbl, "magnitude":dbl[]})
            }
          }
        }
        n2004 = case shown="True" w3705 {
          tunnel: w3706 -> [w3737 w3743]
          tunnel: [w3737 w3738] -> w3704
          frame False {
          }
          frame True {
            n2005 = Array Subset(array=w3743, index (row)=0 ("index"), length (row)=4 ("length"), index (col)=0 ("index"), length (col)=1 ("length")) -> (w3738:T45)
          }
        }
        n2006 = feedback-in #14(w3704) -> ()
        n2007 = Split 1D Array(array=w3718, index=2) -> (first subarray=→"FFT 1":cluster{"f0":dbl, "df":dbl, "magnitude":dbl[]}[], second subarray=→"FFT 2":cluster{"f0":dbl, "df":dbl, "magnitude":dbl[]}[])
      }
    }
    n2008 = case "For plotting results of scanning MCL" shown="True" w2805 {
      tunnel: w2804 -> [_ w3156]
      tunnel: w2720 -> [_ w3252]
      tunnel: w2813 -> [_ _]
      tunnel: w2688 -> [_ w3226]
      tunnel: w2663 -> [_ w3157]
      tunnel: w2662 -> [_ w3130]
      frame False {
      }
      frame True {
        w3137 = u32 0 items=["Horizontal", "Vertical", "Central", "1st Diagonal", "2nd Diagonal"] ("Type of Symmetry")
        w3165 = u32 0 items=["Horizontal", "Vertical", "Central", "1st Diagonal", "2nd Diagonal"] ("Type of Symmetry")
        w3168 = u32 0 items=["Horizontal", "Vertical", "Central", "1st Diagonal", "2nd Diagonal"] ("Type of Symmetry")
        w3197 = u32 0 items=["Horizontal", "Vertical", "Central", "1st Diagonal", "2nd Diagonal"] ("Type of Symmetry")
        n2009 = Index Array(array=w3226, index=10) -> (element=w3232:waveform(dbl))
        n2010 = Index Array(array=w3226, index=11) -> (element=w3229:waveform(dbl))
        n2011 = local read "Cycles/step (MCL)"() -> (w3182:u64)
        n2012 = Index Array(array=w3226, index="Channel") -> (element=w3228:waveform(dbl))
        n2013 = Unbundle(w3130) -> ("New Image"=w3129:T2, "New Image"=w3128:T2, "New Image"=w3127:T2, "New Image"=w3126:T2)
        n2014 = Unbundle By Name(w3232) -> ("Y"=w3184:dbl[])
        n2015 = Unbundle By Name(w3229) -> ("Y"=w3186:dbl[])
        n2016 = Unbundle By Name(w3228) -> ("Y"=w3191:dbl[])
        n2017 = call "downsample 1D array - double.vi"("Ave N"=w3182, "Array In"=w3184) -> ("Array Out"=w3183:dbl[])  [unwired: 1 out]
        n2018 = call "downsample 1D array - double.vi"("Ave N"=w3182, "Array In"=w3186) -> ("Array Out"=w3185:dbl[])  [unwired: 1 out]
        n2019 = call "downsample 1D array - double.vi"("Ave N"=w3182, "Array In"=w3191) -> ("Array Out"=w3190:dbl[])  [unwired: 1 out]
        n2020 = feedback #15(w3252) -> (w3253:dbl[])
        n2021 = Build Array (concatenate)(w3253, w3252) -> (w3234:dbl[])
        n2022 = feedback #16(w3157) -> (w3159:dbl[])
        n2023 = Build Array (concatenate)(w3159, w3157) -> (w3158:dbl[])
        n2024 = local read "Scan steps (MCL)"() -> (w3139:u64)
        n2025 = Select(t=w3252, s=w3156, f=w3234) -> (s? t:f=w3238:dbl[])
        n2026 = feedback-in #15(w3238) -> ()
        n2027 = Select(t=w3157, s=w3156, f=w3158) -> (s? t:f=w3140:dbl[])
        n2028 = feedback-in #16(w3140) -> ()
        n2029 = local read "Scan lines (y)"() -> (w3125:u64)
        n2030 = local read "N APD Samp/step"() -> (w3141:dbl)
        n2031 = feedback #17(w3183) -> (w3240:dbl[])
        n2032 = Build Array (concatenate)(w3240, w3183) -> (w3231:dbl[])
        n2033 = feedback #18(w3190) -> (w3250:dbl[])
        n2034 = Build Array (concatenate)(w3250, w3190) -> (w3249:dbl[])
        n2035 = feedback #19(w3185) -> (w3242:dbl[])
        n2036 = Build Array (concatenate)(w3242, w3185) -> (w3243:dbl[])
        n2037 = Select(t=w3183, s=w3156, f=w3231) -> (s? t:f=w3187:dbl[])
        n2038 = feedback-in #17(w3187) -> ()
        n2039 = Select(t=w3190, s=w3156, f=w3249) -> (s? t:f=w3189:dbl[])
        n2040 = feedback-in #18(w3189) -> ()
        n2041 = Select(t=w3185, s=w3156, f=w3243) -> (s? t:f=w3188:dbl[])
        n2042 = feedback-in #19(w3188) -> ()
        n2043 = Multiply(x=w3139, y=u64 2) -> (x*y=w3124:u64)
        n2044 = call "integrate 1D array interval - double.vi"("Ave N"=w3141, "Array In"=w3140) -> ("Array Out"=w3152:dbl[])  [unwired: 1 out]
        n2045 = call "integrate 1D array interval - double.vi"("Ave N"=w3141, "Array In"=w3238) -> ("Array Out"=w3237:dbl[])  [unwired: 1 out]
        n2046 = Array Size(array=w3152) -> (size(s)=w3153:i32)
        n2047 = Array Size(array=w3237) -> (size(s)=w3239:i32)
        n2048 = Multiply(x=w3125, y=w3124) -> (x*y=w3155:u64)
        n2049 = Multiply(x=w3125, y=w3124) -> (x*y=w3247:u64)
        n2050 = call <vilib>:"Mean.vi"("X"=w3187) -> ("mean"=w3171:dbl)  [unwired: 1 out]
        n2051 = Subtract(x=w3155, y=w3153) -> (x-y=w3146:u64)
        n2052 = call <vilib>:"Mean.vi"("X"=w3189) -> ("mean"=w3176:dbl)  [unwired: 1 out]
        n2053 = call <vilib>:"Mean.vi"("X"=w3188) -> ("mean"=w3174:dbl)  [unwired: 1 out]
        n2054 = call <vilib>:"Mean.vi"("X"=w3152) -> ("mean"=w3143:dbl)  [unwired: 1 out]
        n2055 = Subtract(x=w3247, y=w3239) -> (x-y=w3181:u64)
        n2056 = call <vilib>:"Mean.vi"("X"=w3237) -> ("mean"=w3178:dbl)  [unwired: 1 out]
        n2057 = Initialize Array(1.0 ("element"), w3146) -> (w3142:dbl[])
        n2058 = Initialize Array(1.0 ("element"), w3181) -> (w3172:dbl[])
        n2059 = Multiply(x=w3142, y=w3143) -> (x*y=w3144:dbl[])
        n2060 = Multiply(x=w3172, y=w3174) -> (x*y=w3175:dbl[])
        n2061 = Multiply(x=w3172, y=w3176) -> (x*y=w3177:dbl[])
        n2062 = Multiply(x=w3172, y=w3171) -> (x*y=w3173:dbl[])
        n2063 = Multiply(x=w3172, y=w3178) -> (x*y=w3179:dbl[])
        n2064 = Build Array (concatenate)(w3187, w3173) -> (w3241:dbl[])
        n2065 = Build Array (concatenate)(w3189, w3177) -> (w3245:dbl[])
        n2066 = Build Array (concatenate)(w3188, w3175) -> (w3244:dbl[])
        n2067 = Build Array (concatenate)(w3152, w3144) -> (w3154:dbl[])
        n2068 = Build Array (concatenate)(w3237, w3179) -> (w3246:dbl[])
        n2069 = Reshape Array(w3241, w3125, w3124) -> (w3207:dbl[][])
        n2070 = Reshape Array(w3154, w3125, w3124) -> (w3150:dbl[][])
        n2071 = Reshape Array(w3245, w3125, w3124) -> (w3199:dbl[][])
        n2072 = Reshape Array(w3244, w3125, w3124) -> (w3214:dbl[][])
        n2073 = Reshape Array(w3246, w3125, w3124) -> (w3224:dbl[][])
        n2074 = Array Subset(array=w3214, index (col)=0 ("index"), length (col)=w3139) -> (w3219:dbl[][])  [unwired: 2 in]
        n2075 = Array Subset(array=w3214, index (col)=w3139) -> (w3217:dbl[][])  [unwired: 3 in]
        n2076 = Array Subset(array=w3199, index (col)=0 ("index"), length (col)=w3139) -> (w3205:dbl[][])  [unwired: 2 in]
        n2077 = Array Subset(array=w3199, index (col)=w3139) -> (w3203:dbl[][])  [unwired: 3 in]
        n2078 = Array Subset(array=w3150, index (col)=0 ("index"), length (col)=w3139) -> (w3149:dbl[][])  [unwired: 2 in]
        n2079 = Array Subset(array=w3150, index (col)=w3139) -> (w3147:dbl[][])  [unwired: 3 in]
        n2080 = Array Subset(array=w3224, index (col)=0 ("index"), length (col)=w3139) -> (w3223:dbl[][])  [unwired: 2 in]
        n2081 = Array Subset(array=w3224, index (col)=w3139) -> (w3221:dbl[][])  [unwired: 3 in]
        n2082 = Array Subset(array=w3207, index (col)=0 ("index"), length (col)=w3139) -> (w3212:dbl[][])  [unwired: 2 in]
        n2083 = Array Subset(array=w3207, index (col)=w3139) -> (w3210:dbl[][])  [unwired: 3 in]
        n2084 = for {
          tunnel: w3219 -> [w3261] mode=indexing
          tunnel: [w3260] -> w3218 mode=indexing
          workers-P: _ -> [_]
          n2085 = Reverse 1D Array(array=w3261) -> (reversed array=w3260:dbl[])
        }
        n2086 = for {
          tunnel: w3205 -> [w3257] mode=indexing
          tunnel: [w3256] -> w3204 mode=indexing
          workers-P: _ -> [_]
          n2087 = Reverse 1D Array(array=w3257) -> (reversed array=w3256:dbl[])
        }
        n2088 = for {
          tunnel: w3149 -> [w3255] mode=indexing
          tunnel: [w3254] -> w3148 mode=indexing
          workers-P: _ -> [_]
          n2089 = Reverse 1D Array(array=w3255) -> (reversed array=w3254:dbl[])
        }
        n2090 = for {
          tunnel: w3223 -> [w3263] mode=indexing
          tunnel: [w3262] -> w3222 mode=indexing
          workers-P: _ -> [_]
          n2091 = Reverse 1D Array(array=w3263) -> (reversed array=w3262:dbl[])
        }
        n2092 = for {
          tunnel: w3212 -> [w3259] mode=indexing
          tunnel: [w3258] -> w3211 mode=indexing
          workers-P: _ -> [_]
          n2093 = Reverse 1D Array(array=w3259) -> (reversed array=w3258:dbl[])
        }
        n2094 = Index Array(array=w3224, index (row)=0) -> (element=→"Waveform Graph":dbl[])  [unwired: 1 in]
        n2095 = Add(x=w3218, y=w3217) -> (x+y=w3216:dbl[][])
        n2096 = Add(x=w3204, y=w3203) -> (x+y=w3202:dbl[][])
        n2097 = Add(x=w3148, y=w3147) -> (x+y=w3132:dbl[][])
        n2098 = Add(x=w3222, y=w3221) -> (x+y=w3196:dbl[][])
        n2099 = Add(x=w3211, y=w3210) -> (x+y=w3209:dbl[][])
        n2100 = Divide(x=w3202, y=2) -> (x/y=w3200:dbl[][])
        n2101 = Divide(x=w3216, y=2) -> (x/y=w3161:dbl[][])
        n2102 = Divide(x=w3209, y=2) -> (x/y=w3163:dbl[][])
        n2103 = To Single Precision Float(number=w3196) -> (single precision float=w3195:sgl[][])
        n2104 = Transpose 2D Array(2D array=w3200) -> (transposed array=→"Data map":dbl[][])
        n2105 = To Single Precision Float(number=w3132) -> (single precision float=w3136:sgl[][])
        n2106 = To Single Precision Float(number=w3161) -> (single precision float=w3167:sgl[][])
        n2107 = To Single Precision Float(number=w3163) -> (single precision float=w3164:sgl[][])
        n2108 = call "IMAQ ArrayToImage"("Image Pixels (Float)"=w3195, "Image"=w3129) -> ("Image Out"=w3198:T2)  [unwired: 8 in, 1 out]
        n2109 = call "IMAQ ArrayToImage"("Image Pixels (Float)"=w3136, "Image"=w3128) -> ("Image Out"=w3138:T2)  [unwired: 8 in, 1 out]
        n2110 = call "IMAQ ArrayToImage"("Image Pixels (Float)"=w3167, "Image"=w3127) -> ("Image Out"=w3169:T2)  [unwired: 8 in, 1 out]
        n2111 = call "IMAQ ArrayToImage"("Image Pixels (Float)"=w3164, "Image"=w3126) -> ("Image Out"=w3166:T2)  [unwired: 8 in, 1 out]
        n2112 = call "IMAQ Symmetry"("Type of Symmetry"=w3197, "Image Src"=w3198) -> ("Image Dst Out"=w3193:T2)  [unwired: 3 in, 1 out]
        n2113 = call "IMAQ Symmetry"("Type of Symmetry"=w3137, "Image Src"=w3138) -> ("Image Dst Out"=w3134:T2)  [unwired: 3 in, 1 out]
        n2114 = call "IMAQ Symmetry"("Type of Symmetry"=w3168, "Image Src"=w3169) -> ("Image Dst Out"=→"Detection Laser X":T2)  [unwired: 3 in, 1 out]
        n2115 = call "IMAQ Symmetry"("Type of Symmetry"=w3165, "Image Src"=w3166) -> ("Image Dst Out"=→"Detection Laser Y":T2)  [unwired: 3 in, 1 out]
        n2116 = call "IMAQ Set Simple Calibration"("Calibration Axis Info"=T35 {"Origin Pixel"={"X"=0.0, "Y"=0.0}, "Angle Relative to Horizontal (deg)"=0.0, "Axis Reference"=0}, "Grid Descriptor"=T36 {"X Step"=0.3, "Y Step"=0.3, "Unit"=enum."Undefined"}, "Image"=w3193) -> ("Calibrated Image"=→"APD 1":T2)  [unwired: 7 in, 1 out]
        n2117 = call "IMAQ Set Simple Calibration"("Calibration Axis Info"=T35 {"Origin Pixel"={"X"=0.0, "Y"=0.0}, "Angle Relative to Horizontal (deg)"=0.0, "Axis Reference"=0}, "Grid Descriptor"=T36 {"X Step"=0.3, "Y Step"=0.3, "Unit"=enum."Undefined"}, "Image"=w3134) -> ("Calibrated Image"=→"APD 2":T2)  [unwired: 7 in, 1 out]
      }
    }
    n2118 = Subtract(x=w2669, y="APD 2 Offset") -> (x-y=w2666:waveform(dbl))
    n2119 = Subtract(x=w2671, y="APD 1 Offset") -> (x-y=w2667:waveform(dbl))
    n2120 = Index Array(array=w2686, index=3) -> (element=w2749:waveform(dbl))
    n2121 = Index Array(array=w2686, index=6) -> (element=w2746:waveform(dbl))
    n2122 = Build Array(w2667, w2666) -> (→"APD Chart":waveform(dbl)[])
    n2123 = Array Size(array=w2738) -> (size(s)=w2793:i32)
    n2124 = call <vilib>:"Std Deviation and Variance.vi"("X"=w2679) -> ("standard deviation"=w2678:dbl)  [unwired: 1 in, 2 out]
    n2125 = Add Array Elements(numeric array=w2679) -> (sum=w2681:u32)
    n2126 = Add Array Elements(numeric array=w2738) -> (sum=w2803:u32)
    n2127 = call <vilib>:"Std Deviation and Variance.vi"("X"=w2738) -> ("standard deviation"=w2737:dbl)  [unwired: 1 in, 2 out]
    n2128 = Divide(x="T1 offset_x (mV)", y=1000.0) -> (x/y=w2750:dbl)
    n2129 = Divide(x=w2678, y=w2677) -> (x/y=w2674:dbl)
    "Rate sigma (Hz) 2" <- w2674
    n2130 = Multiply(x=w2677, y=w2793) -> (x*y=w2680:dbl)
    "Int. Time (s)" <- w2680
    n2131 = Divide(x=w2681, y=w2680) -> (x/y=w2675:dbl)
    "APD 2 Rate (Hz)" <- w2675
    n2132 = Divide(x=w2803, y=w2680) -> (x/y=w2735:dbl)
    "APD 1 Rate (Hz)" <- w2735
    n2133 = Divide(x=w2737, y=w2677) -> (x/y=w2736:dbl)
    "Rate sigma (Hz)" <- w2736
    n2134 = Divide(x=w2674, y=w2675) -> (x/y=→"Sigma/Mean 2":dbl)
    n2135 = Divide(x=w2736, y=w2735) -> (x/y=→"Sigma/Mean":dbl)
    n2136 = feedback-in #20("Calibration") -> ()
    n2137 = feedback #20(u16 1 ("Calibration")) -> (w2770:u16)
    n2138 = Divide(x="T2 offset_x (mV)", y=1000.0) -> (x/y=w2748:dbl)
    n2139 = case shown="0, Default" "Calibration" {
      tunnel: "T1 alpha_x (nm/V)" -> [_ w3092 w3113]
      tunnel: "T1 kappa_x (pN/nm)" -> [_ _ w3103]
      tunnel: "T2 alpha_x (nm/V)" -> [_ w3091 w3111]
      tunnel: "T2 kappa_x (pN/nm)" -> [_ _ w3104]
      tunnel: w2749 -> [w3074 w3089 w3109]
      tunnel: w2746 -> [w3073 w3087 w3107]
      tunnel: [w3074 w3086 w3106] -> w2779
      tunnel: [w3073 w3085 w3105] -> w2778
      tunnel: ["T1 X (V)" ("Label.Text") "T1 X (nm)" ("Label.Text") "T1 X (pN)" ("Label.Text")] -> w2767
      tunnel: ["T2 X (V)" ("Label.Text") "T2 X (nm)" ("Label.Text") "T2 X (pN)" ("Label.Text")] -> w2766
      tunnel: ["Position (V)" ("Label.Text") "Position (nm)" ("Label.Text") "Force (pN)" ("Label.Text")] -> w2768
      tunnel: w2748 -> [_ w3077 w3096]
      tunnel: w2750 -> [_ w3080 w3098]
      tunnel: ["Mean (V)" ("Label.Text") "Mean (nm)" ("Label.Text") "Mean (pN)" ("Label.Text")] -> w2763
      tunnel: ["Difference (V)" ("Label.Text") "Difference (nm)" ("Label.Text") "Difference (pN)" ("Label.Text")] -> w2694
      frame 0, Default {
      }
      frame 1 {
        n2140 = Unbundle By Name(w3089) -> ("Y"=w3093:dbl[])
        n2141 = Unbundle By Name(w3087) -> ("Y"=w3078:dbl[])
        n2142 = Subtract(x=w3093, y=w3080) -> (x-y=w3081:dbl[])
        n2143 = Subtract(x=w3078, y=w3077) -> (x-y=w3079:dbl[])
        n2144 = Multiply(x=w3079, y=w3091) -> (x*y=w3088:dbl[])
        n2145 = Multiply(x=w3092, y=w3081) -> (x*y=w3090:dbl[])
        n2146 = Bundle By Name(cluster=w3087, "Y"=w3088) -> (w3085:waveform(dbl))
        n2147 = Bundle By Name(cluster=w3089, "Y"=w3090) -> (w3086:waveform(dbl))
      }
      frame 2 {
        n2148 = Unbundle By Name(w3109) -> ("Y"=w3114:dbl[])
        n2149 = Unbundle By Name(w3107) -> ("Y"=w3112:dbl[])
        n2150 = Subtract(x=w3112, y=w3096) -> (x-y=w3097:dbl[])
        n2151 = Subtract(x=w3114, y=w3098) -> (x-y=w3099:dbl[])
        n2152 = Compound Arithmetic op=MULTIPLY(w3097, w3111, w3104) -> (w3108:dbl[])
        n2153 = Compound Arithmetic op=MULTIPLY(w3103, w3113, w3099) -> (w3110:dbl[])
        n2154 = Bundle By Name(cluster=w3107, "Y"=w3108) -> (w3105:waveform(dbl))
        n2155 = Bundle By Name(cluster=w3109, "Y"=w3110) -> (w3106:waveform(dbl))
      }
    }
    n2156 = Not Equal?(x=w2770, y="Calibration") -> (x != y?=w2725:bool)
    n2157 = case shown="True" w2725 {
      tunnel: w2768 -> [_ w3067]
      tunnel: w2767 -> [_ w3066]
      tunnel: w2766 -> [_ w3065]
      tunnel: w2763 -> [_ w3064]
      tunnel: w2694 -> [_ w3063]
      frame False {
      }
      frame True {
        n2158 = property on="Force" class="WFChart (strict)"("YScale.NameLbl.Text"=w3067) -> ()  [unwired: 2 in, 2 out]
        n2159 = property on="T2 X" class="DigNum (strict)"("Caption.Text"=w3065) -> ()  [unwired: 2 in, 2 out]
        n2160 = property on="T1 X" class="DigNum (strict)"("Caption.Text"=w3066) -> ()  [unwired: 2 in, 2 out]
        n2161 = property on="Mean" class="DigNum (strict)"("Caption.Text"=w3064) -> ()  [unwired: 2 in, 2 out]
        n2162 = property on="Difference" class="DigNum (strict)"("Caption.Text"=w3063) -> ()  [unwired: 2 in, 2 out]
      }
    }
    n2163 = Unbundle By Name(w2749) -> ("Y"=w2752:dbl[])
    n2164 = Unbundle By Name(w2746) -> ("Y"=w2755:dbl[])
    n2165 = Subtract(x=w2752, y=w2750) -> (x-y=w2753:dbl[])
    n2166 = Subtract(x=w2755, y=w2748) -> (x-y=w2754:dbl[])
    n2167 = Multiply(x=w2754, y="T2 alpha_x (nm/V)") -> (x*y=w2745:dbl[])
    n2168 = Multiply(x="T1 alpha_x (nm/V)", y=w2753) -> (x*y=w2744:dbl[])
    n2169 = Not(x="Trap Trig. Fl.") -> (.not. x?=w2573:bool)
    n2170 = Multiply(x=w2778, y=-1.0) -> (x*y=w2757:waveform(dbl))
    n2171 = Subtract(x=w2745, y=w2744) -> (x-y=w2743:dbl[])
    n2172 = Unbundle By Name(w2778) -> ("Y"=w2714:dbl[])
    n2173 = Unbundle By Name(w2779) -> ("Y"=w2537:dbl[])
    n2174 = Build Array(w2779, w2757) -> (→"Force":waveform(dbl)[])
    n2175 = Subtract(x=w2743, y="Offset (nm)") -> (x-y=w2712:dbl[])
    n2176 = case shown="True" "Read Lateness and Rel Phase" {
      tunnel: w2553 -> [w3040 w3062]
      tunnel: w2552 -> [w3041 w3061]
